vi "Enclose with Diagram Disable Structure.vi"(8 "Error In":errorcluster) -> (0 "Error Out":errorcluster)   [LabVIEW 2018, in "Tests.lvlib" / "Toolkit.lvlib" / "Unit.lvlib"]
uses:
  Unit.lvlib
  <vilib>/addons/_JKI Toolkits/Caraya/classes/Test/Test.lvclass
  <vilib>/Utility/traverseref.llb/VI Scripting - Traverse.lvlib
  <vilib>/Utility/traverseref.llb/TRef TravTarget.ctl
  <vilib>/addons/_JKI Toolkits/Caraya/classes/Assert/Assert.lvclass
  src/Toolkit/Toolkit.lvlib
  Tests.lvlib
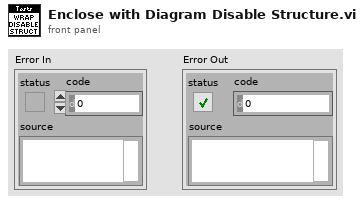
[diagram p1: front panel]
types:
  T1 = typedef "TRef TravTarget.ctl" = enum16{"FP", "BD", "Other"}
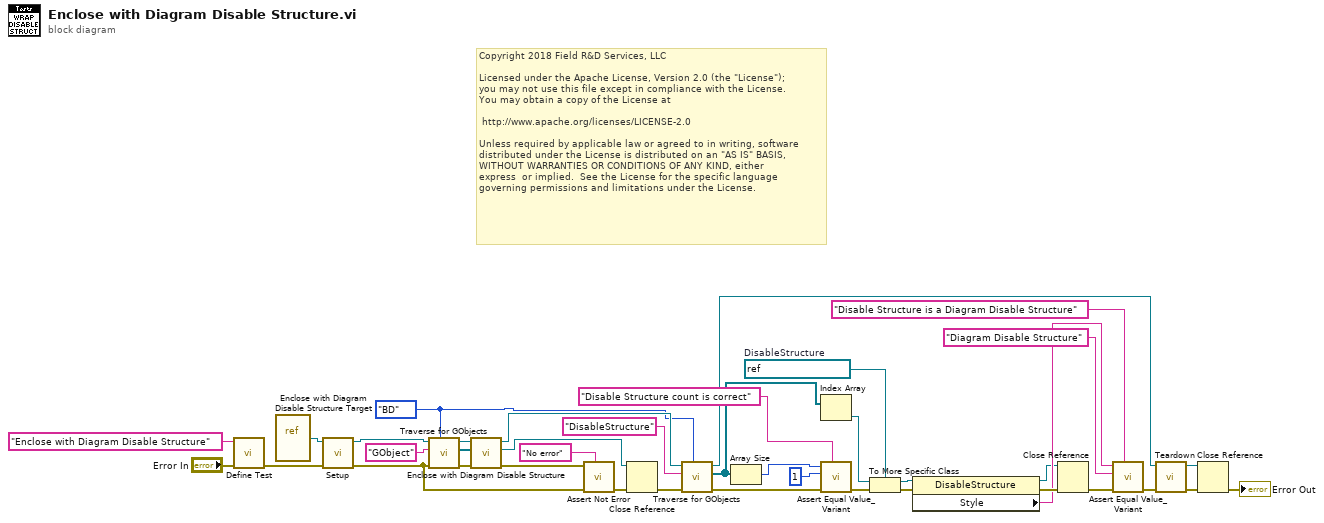
[diagram p0: block diagram]
diagram:
  w6 = refnum<vi> refnum  # DisableStructure
  w13 = TRef_TravTarget."BD" ("Traverse Target")
  # "Copyright 2018 Field R&D Services, LLC\n\nLicensed under the Apache License, Version 2.0 (the \"License\");\nyou may not use this file except in compliance with the License.\nYou may obtain a copy of the License at\n\n\thttp://www.apache.org/licenses/LICENSE-2.0\n\nUnless required by applicable law or agreed to in writing, software\ndistributed under the License is distributed on an \"AS IS\" BASIS,\nWITHOUT WARRANTIES OR CONDITIONS OF ANY KIND, either \nexpress  or implied.  See the License for the specific language \ngoverning permissions and limitations under the License."
  n1 = call <vilib>:"Define Test.vi"("error in (no error)"="Error In", "Label (VI Title)"="Enclose with Diagram Disable Structure") -> ("error out"=w30:errorcluster)  [unwired: 9 in]
  n2 = vi-ref "Enclose with Diagram Disable Structure Target.vi"() -> (w35:refnum<vi>)
  n3 = call "Setup.vi"("Error In"=w30, "VI In"=w35) -> ("Error Out"=w27:errorcluster, "VI Out"=w34:refnum<vi>)  [unwired: 8 in]
  n4 = call <vilib>:"Traverse for GObjects.vi"("Traverse Target"=w13, "error in (no error)"=w27, "Class Name"="GObject", "VI Refnum"=w34) -> ("error out"=w36:errorcluster, "References"=w17:refnum<vi>[], "dup VI Refnum"=w18:refnum<vi>)  [unwired: 4 in, 1 out]
  n5 = call "Enclose with Diagram Disable Structure.vi"("Error In"=w36, "Selection List[]"=w17, "VI In"=w18) -> ("Error Out"=w25:errorcluster, "Structure"=w31:refnum<vi>, "VI Out"=w15:refnum<vi>)  [unwired: 6 in]
  n6 = call <vilib>:"Assert Not Error.vi"("Label"="No error", "error in (no error)"=w27, "Not Error?"=w25) -> ("error out"=w26:errorcluster)  [unwired: 8 in]
  n7 = Close Reference(reference=w31, error in (no error)=w26) -> (error out=w16:errorcluster)
  n8 = call <vilib>:"Traverse for GObjects.vi"("Traverse Target"=w13, "error in (no error)"=w16, "Class Name"="DisableStructure", "VI Refnum"=w15) -> ("error out"=w11:errorcluster, "References"=w10:refnum<vi>[], "dup VI Refnum"=w14:refnum<vi>)  [unwired: 4 in, 1 out]
  n9 = Array Size(array=w10) -> (size(s)=w22:i32)
  n10 = Index Array(array=w10) -> (element=w7:refnum<vi>)  [unwired: 1 in]
  n11 = call <vilib>:"Assert Equal Value_Variant.vi"("Label"="Disable Structure count is correct", "error in (no error)"=w11, "Y"=1 ("size(s)"), "X"=w22) -> ("error out"=w19:errorcluster)  [unwired: 7 in]
  n12 = To More Specific Class(target class=w6, reference=w7, error in=w19) -> (specific class reference=w5:refnum<vi>, error out=w8:errorcluster)
  n13 = property class="DisableStructure"(reference=w5, error in=w8) -> (reference out=w2:refnum<vi>, error out=w9:errorcluster, "Style"=w4:string)
  n14 = Close Reference(reference=w2, error in (no error)=w9) -> (error out=w3:errorcluster)
  n15 = call <vilib>:"Assert Equal Value_Variant.vi"("Label"="Disable Structure is a Diagram Disable Structure", "error in (no error)"=w3, "Y"="Diagram Disable Structure", "X"=w4) -> ("error out"=w28:errorcluster)  [unwired: 7 in]
  n16 = call "Teardown.vi"("Error In"=w28, "VI In"=w14) -> ("Error Out"=w32:errorcluster, "VI Out"=w33:refnum<vi>)  [unwired: 8 in]
  n17 = Close Reference(reference=w33, error in (no error)=w32) -> (error out=→"Error Out":errorcluster)
